vi "close device.vi"(8 "error in (no error)":errorcluster, 11 "Device in":T1) -> (0 "error out":errorcluster, 3 "Device out":T1)   [LabVIEW 2015]
uses:
  typedefs/device.ctl
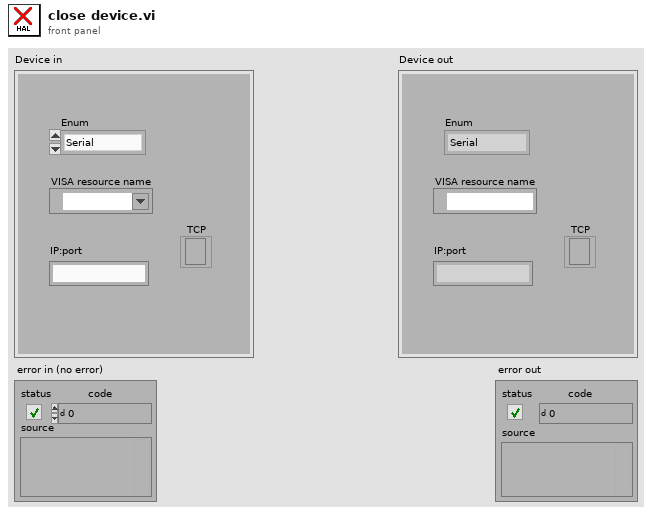
[diagram p1: front panel]
types:
  T1 = typedef "device.ctl" = cluster{"Enum":enum16{"Serial", "TCP/IP", "Mock"}, "IP:port":string, "VISA resource name":refnum<visa-resource-name>, "TCP":refnum<k5>}
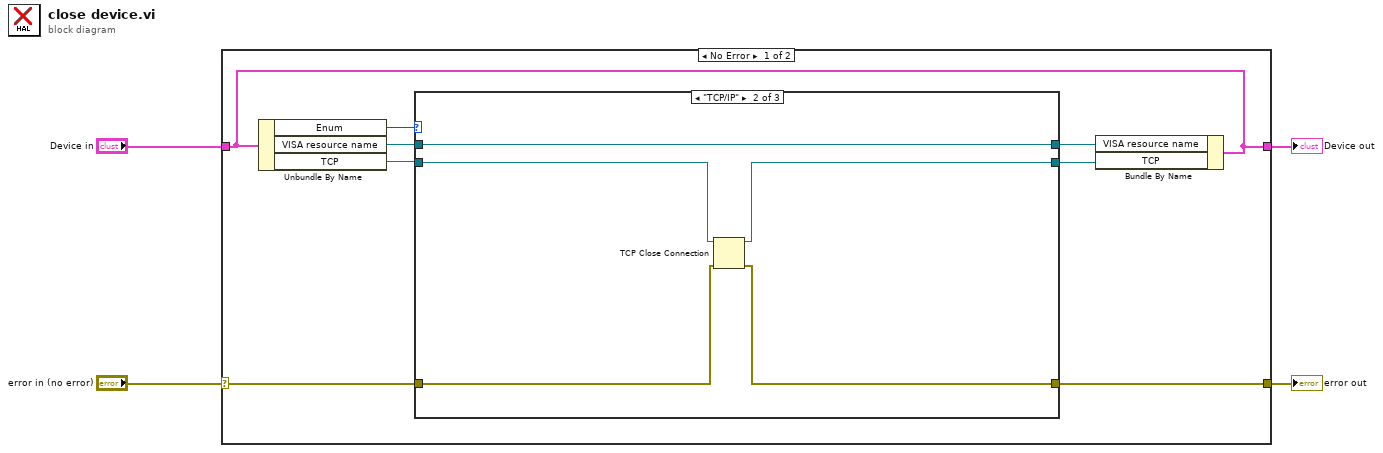
[diagram p0: block diagram]
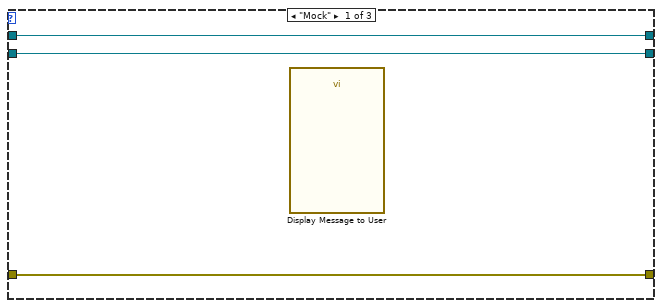
[diagram p2: hidden frame]
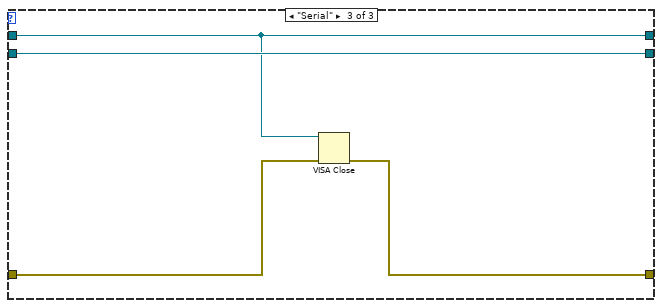
[diagram p3: hidden frame]
diagram:
  n1 = case shown="No Error" "error in (no error)" {
    selector: "error in (no error)" -> [w12 w25]
    tunnel: [w5 w26] -> w3
    tunnel: "Device in" -> [w5 w26]
    tunnel: [w11 w25] -> w1
    frame No Error {
      n2 = Unbundle By Name(w5) -> ("Enum"=w8:enum16{"Serial", "TCP/IP", "Mock"}, "VISA resource name"=w9:refnum<visa-resource-name>, "TCP"=w10:refnum<k5>)
      n3 = case shown="\"TCP/IP\"" w8 {
        tunnel: w10 -> [w15 w19 w24]
        tunnel: w9 -> [w14 w20 w21]
        tunnel: w12 -> [w13 w17 w23]
        tunnel: [w13 w16 w22] -> w11
        tunnel: [w15 w18 w24] -> w7
        tunnel: [w14 w20 w21] -> w6
        frame "Mock" {
          n4 = call "Display Message to User"() -> ()  [unwired: 10 in, 2 out]
        }
        frame "TCP/IP" {
          n5 = TCP Close Connection(connection ID=w19, error in (no error)=w17) -> (connection ID out=w18:refnum<k5>, error out=w16:errorcluster)  [unwired: 1 in]
        }
        frame "Serial" {
          n6 = VISA Close(VISA resource name=w21, error in (no error)=w23) -> (error out=w22:errorcluster)
        }
      }
      n7 = Bundle By Name(cluster=w5, "VISA resource name"=w6, "TCP"=w7) -> ()  [unwired: 1 out]
    }
    frame Error {
    }
  }
  "error out" <- w1
  "Device out" <- w3
